vi "Create Append Group.vi"(8 "error in":errorcluster, 11 "TDMS in":refnum<class "TDMS.lvclass">) -> (0 "error out":errorcluster, 3 "TDMS out":refnum<class "TDMS.lvclass">)   [LabVIEW 2019, in "TDMS.lvlib" / "TDMS.lvclass"]
uses:
  TDMS.lvclass
  TDMS.lvclass/TDMS.ctl
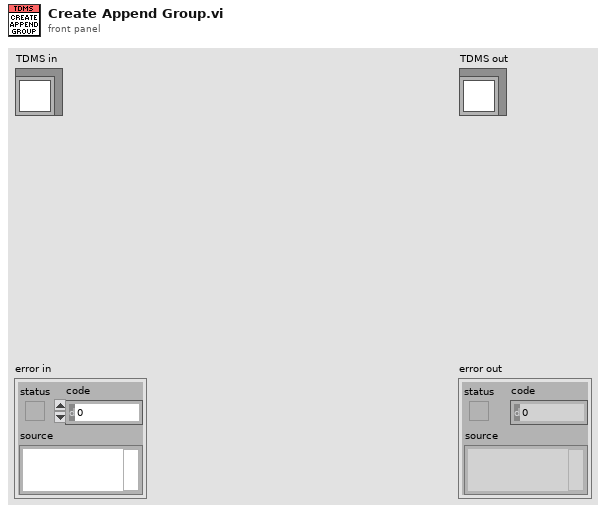
[diagram p1: front panel]
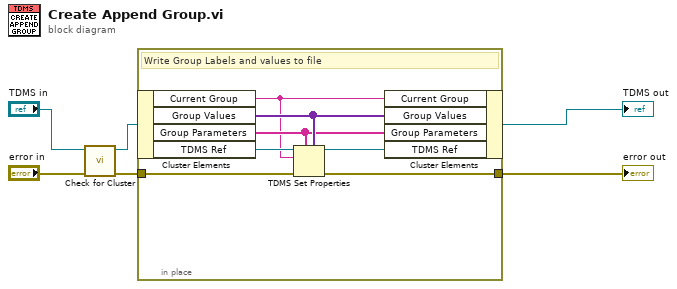
[diagram p0: block diagram]
diagram:
  n1 = call "Check for Cluster.vi"("error in (no error)"="error in", "TDMS in"="TDMS in") -> ("error out"=w1:errorcluster, "TDMS out"=w3:refnum<class "TDMS.lvclass">)  [unwired: 8 in]
  n2 = in-place {
    in-place-border: [w11] -> w5
    in-place-border: w1 -> [w10]
    # "Write Group Labels and values to file"
    n3 = in-place-cluster #1(w3) -> ("Current Group"=w7:string, "Group Values"=w9:variant[], "Group Parameters"=w8:string[], "TDMS Ref"=w13:refnum<k34>)
    n4 = TDMS Set Properties(5:w9, 7:w8, 8:w10, 10:w7, 11:w13) -> (0:w11:errorcluster, 3:w12:refnum<k34>)  [unwired: 1 in, 2 out]
    n5 = in-place-cluster #1("Current Group"=w7, "Group Values"=w9, "Group Parameters"=w8, "TDMS Ref"=w12) -> (→"TDMS out":refnum<class "TDMS.lvclass">)
  }
  "error out" <- w5
